vi "read serial reply.vi"(8 "error in (no error)":errorcluster, 11 "Serial Port":refnum<visa-resource-name>) -> (0 "error out":errorcluster, 2 "reply":string, 3 "Serial Port out":refnum<visa-resource-name>)   [LabVIEW 2012]
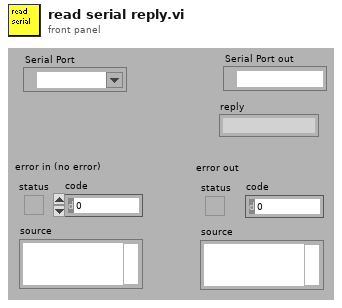
[diagram p1: front panel]
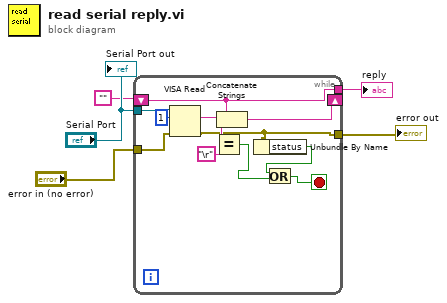
[diagram p0: block diagram]
diagram:
  n1 = while {
    tunnel: "Serial Port" -> [w16]
    shift-right: [w14] -> _
    shift-left: "" -> [w11]
    tunnel: [w11] -> w4
    tunnel: "error in (no error)" -> [w10]
    tunnel: [w9] -> w5
    stop <- w8 stop-if-true
    n2 = VISA Read(VISA resource name=w16, byte count=u32 1, error in (no error)=w10) -> (read buffer=w13:string, error out=w9:errorcluster)  [unwired: 2 out]
    n3 = Equal?(x=w13, y="\r") -> (x = y?=w7:bool)
    n4 = Concatenate Strings(w11, w13) -> (w14:string)
    n5 = Unbundle By Name(w9) -> ("status"=w6:bool)
    n6 = Or(x=w6, y=w7) -> (x .or. y?=w8:bool)
  }
  "error out" <- w5
  "reply" <- w4
  "Serial Port out" <- "Serial Port"
